vi "Get System Dependencies.vi"(8 "error in (no error)":errorcluster, 11 "System in":refnum<class "System.lvclass">) -> (0 "error out":errorcluster, 2 "Pump":refnum<class "Pump.lvclass">, 3 "System out":refnum<class "System.lvclass">)   [LabVIEW 2014, in "System.lvclass"]
uses:
  System.lvclass
  Pump class/Pump.lvclass
  <vilib>/JKI/JKI SMO/SMO/Typedefs/Search Key.ctl
  <vilib>/JKI/JKI SMO/SMO/SMO.lvclass
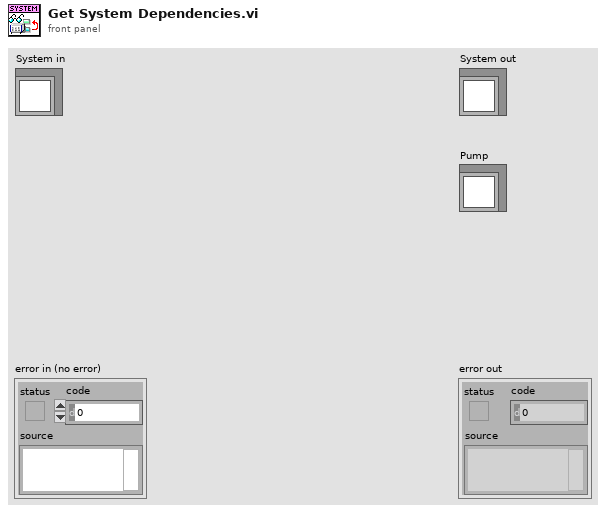
[diagram p1: front panel]
types:
  T1 = typedef "SMO.lvclass/Search Key.ctl" = enum16{"Name", "GUID", "Qualified Name", "Subsystem Path", "Configuration Path"}
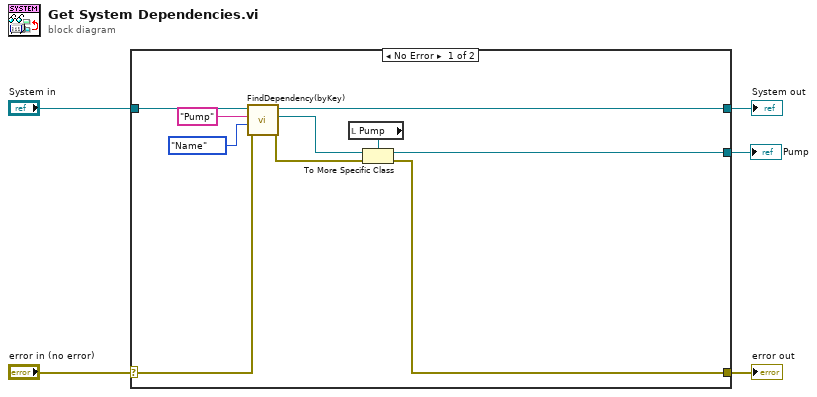
[diagram p0: block diagram]
diagram:
  n1 = case shown="No Error" "error in (no error)" {
    selector: "error in (no error)" -> [w12 w17]
    tunnel: [w6 w17] -> w4
    tunnel: [w11 w16] -> w2
    tunnel: "System in" -> [w15 w16]
    tunnel: [w8 _] -> w1
    frame No Error {
      n2 = call <vilib>:"FindDependency(byKey).vi"("error in (no error)"=w12, "Search Key (Name)"=Search_Key."Name", "Key"="Pump", "SMO in"=w15) -> ("error out"=w7:errorcluster, "Dependency"=w9:refnum<class "SMO.lvclass">, "SMO dup"=w11:refnum<class "System.lvclass">)  [unwired: 4 in, 1 out]
      n3 = local read "Pump"() -> (w10:refnum<class "Pump.lvclass">)
      n4 = To More Specific Class(target class=w10, reference=w9, error in=w7) -> (specific class reference=w8:refnum<class "Pump.lvclass">, error out=w6:errorcluster)
    }
    frame Error {
    }
  }
  "error out" <- w4
  "System out" <- w2
  "Pump" <- w1
